vi "Benchmark mupExpr_eval.vi"(8 "error in (no error)":errorcluster, 10 "Iterations":i32, 11 "Expression":string) -> (0 "error out":errorcluster, 2 "x":dbl[](array[numeric]), 3 "y":dbl[](array[numeric]), 5 "dt average":dbl)   [LabVIEW 2015]
uses:
  mupExpr/mupExpr.lvclass/mupExpr.ctl
  mupLib/mupEval.vi
  mupLib/mupSetVarValue.vi
  mupLib/mupCheckError.vi
  mupLib/mupLibPath.vi
  <vilib>/Utility/error.llb/Error Cluster From Error Code.vi
  mupExpr/mupExpr.lvclass
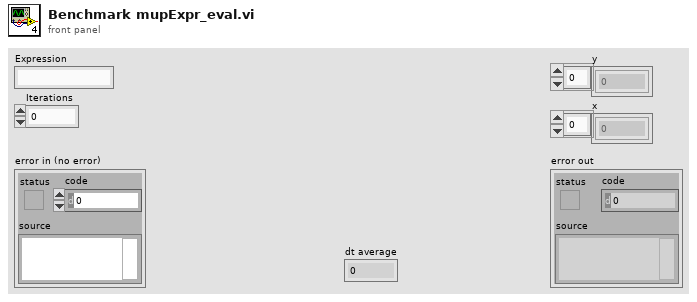
[diagram p1: front panel]
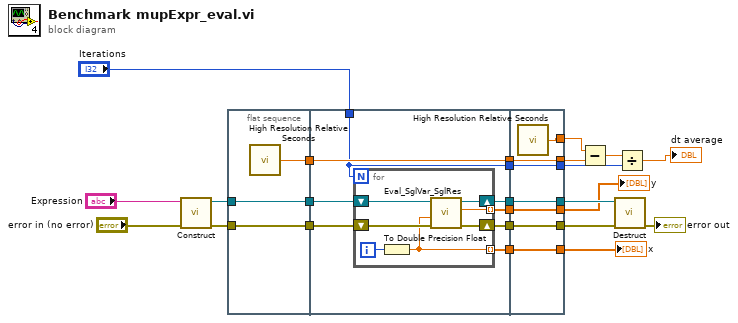
[diagram p0: block diagram]
diagram:
  n1 = call "Construct.vi"("error in (no error)"="error in (no error)", "Expression"="Expression") -> ("error out"=w22:errorcluster, "mupExpr out"=w23:refnum<data-value>)  [unwired: 7 in, 1 out]
  n2 = flat-sequence {
    tunnel: w22 -> [w26]
    tunnel: w23 -> [w27]
    tunnel: [w27] -> w15
    tunnel: [w26] -> w14
    tunnel: [w25] -> w8
    tunnel: w15 -> [w35]
    tunnel: w14 -> [w34]
    tunnel: [w33] -> w13
    tunnel: [w32] -> w12
    tunnel: [w31] -> w11
    tunnel: [w30] -> w10
    tunnel: [w29] -> w9
    tunnel: w8 -> [w29]
    tunnel: "Iterations" -> [w28]
    tunnel: [w28] -> w2
    tunnel: [w46] -> w18
    tunnel: [w47] -> w19
    tunnel: [w48] -> w20
    tunnel: [w49] -> w21
    tunnel: w13 -> [w49]
    tunnel: w12 -> [w48]
    tunnel: w11 -> [w47]
    tunnel: w10 -> [w46]
    tunnel: [w45] -> w6
    tunnel: w9 -> [w45]
    tunnel: [w44] -> w7
    tunnel: [w43] -> w3
    tunnel: w2 -> [w43]
    frame #0 {
      n3 = call <vilib>:"High Resolution Relative Seconds.vi"() -> ("relative seconds"=w25:dbl)
    }
    frame #1 {
      n4 = for {
        N: w28 -> [_]
        shift-right: [w40] -> w32
        shift-left: w34 -> [w41]
        shift-right: [w39] -> w33
        shift-left: w35 -> [w38]
        tunnel: [w37] -> w31 mode=indexing
        tunnel: [w36] -> w30 mode=indexing
        i -> [w42]
        n5 = To Double Precision Float(number=w42) -> (double precision float=w36:dbl)
        n6 = call "Eval_SglVar_SglRes.vi"("error in (no error)"=w41, "varValue"=w36, "mupExpr in"=w38) -> ("error out"=w40:errorcluster, "Result"=w37:dbl, "mupExpr out"=w39:refnum<data-value>)  [unwired: 6 in]
      }
    }
    frame #2 {
      n7 = call <vilib>:"High Resolution Relative Seconds.vi"() -> ("relative seconds"=w44:dbl)
    }
  }
  n8 = Subtract(x=w7, y=w6) -> (x-y=w4:dbl)
  n9 = call "Destruct.vi"("error in (no error)"=w20, "mupExpr in"=w21) -> ("error out"=→"error out":errorcluster)  [unwired: 9 in]
  n10 = Divide(x=w4, y=w3) -> (x/y=→"dt average":dbl)
  "y" <- w19
  "x" <- w18
